vi "Complex Trigger Add Trigger.vi"(7 "Threshold S1/S2":u16(ring) items=["S1", "S2"], 8 "error in (no error)":errorcluster, 9 "Positive or negative (edge or level)":u16(ring) items=["Positive", "Negative"], 10 "Channel":u16(ring) items=["A1", "A2", "A3", "A4", "A5", "A6", "A7", "A8", "A9", "A10", "A11", "A12", "A13", "A14", "A15", "A16", "A17", "A18", "A19", "A20", "B1", "B2", "B3", "B4", "B5", "B6", "B7", "B8", "B9", "B10", "B11", "B12", "B13", "B14", "B15", "B16", "B17", "B18", "B19", "B20", "C1", "C2", "C3", "C4", "C5", "C6", "C7", "C8", "C9", "C10", "C11", "C12", "C13", "C14", "C15", "C16", "C17", "C18", "C19", "C20", "D1", "D2", "D3", "D4", "D5", "D6", "D7", "D8", "D9", "D10", "D11", "D12", "D13", "D14", "D15", "D16", "D17", "D18", "D19", "D20", "E1", "E2", "E3", "E4", "E5", "E6", "E7", "E8", "E9", "E10", "E11", "E12", "E13", "E14", "E15", "E16", "E17", "E18", "E19", "E20", "F1", "F2", "F3", "F4", "F5", "F6", "F7", "F8", "F9", "F10", "F11", "F12", "F13", "F14", "F15", "F16", "F17", "F18", "F19", "F20", "G1", "G2", "G3", "G4", "G5", "G6", "G7", "G8", "G9", "G10", "G11", "G12", "G13", "G14", "G15", "G16", "G17", "G18", "G19", "G20", "H1", "H2", "H3", "H4", "H5", "H6", "H7", "H8", "H9", "H10", "H11", "H12", "H13", "H14", "H15", "H16", "H17", "H18", "H19", "H20", "I1", "I2", "I3", "I4", "I5", "I6", "I7", "I8", "I9", "I10", "I11", "I12", "I13", "I14", "I15", "I16", "I17", "I18", "I19", "I20", "J1", "J2", "J3", "J4", "J5", "J6", "J7", "J8", "J9", "J10", "J11", "J12", "J13", "J14", "J15", "J16", "J17", "J18", "J19", "J20", "K1", "K2", "K3", "K4", "FA1", "FA2", "FA3", "FA4", "FB1", "FB2", "FB3", "FB4", "FC1", "FC2", "FC3", "FC4", "FD1", "FD2", "FD3", "FD4", "FE1", "FE2", "FE3", "FE4", "FF1", "FF2", "FF3", "FF4", "FG1", "FG2", "FG3", "FG4", "FH1", "FH2", "FH3", "FH4", "FI1", "FI2", "FI3", "FI4", "FJ1", "FJ2", "FJ3", "FJ4"], 11 "VISA resource name":refnum<visa-resource-name>) -> (0 "error out":errorcluster, 3 "VISA resource name out":refnum<visa-resource-name>)   [LabVIEW 2017, in "Sefram DAS220.lvlib"]
doc: "Add a trigger condition for complex (multiple) trigger."
uses:
  <instrlib>/Sefram DAS220/Sefram DAS220.lvlib
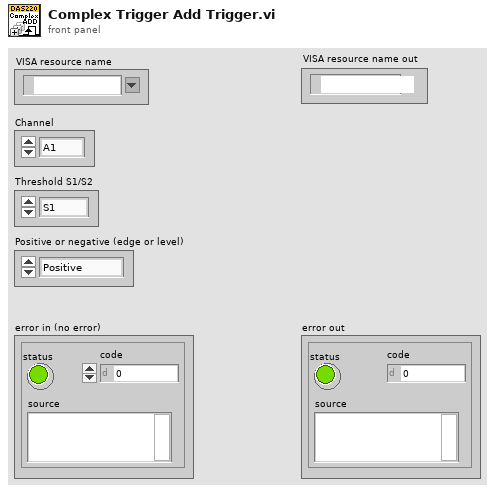
[diagram p1: front panel]
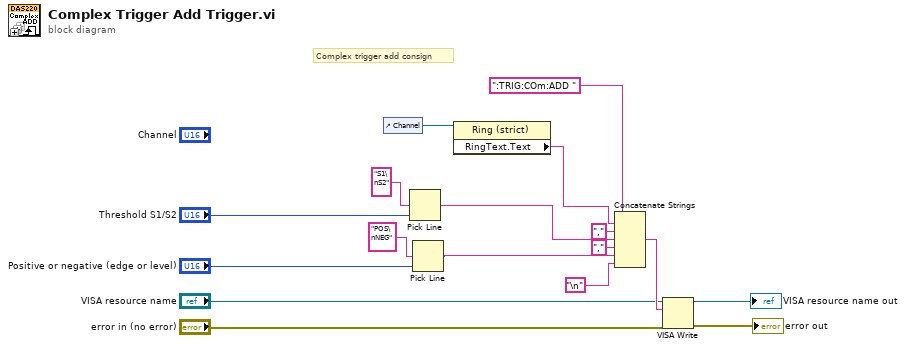
[diagram p0: block diagram]
diagram:
  # "Complex trigger add consign"
  n1 = control-ref of="Channel"() -> (w1:refnum<vi>)
  n2 = Pick Line(multi-line string="S1\nS2", line index="Threshold S1/S2") -> (output string=w7:string)  [unwired: 1 in]
  n3 = Pick Line(multi-line string="POS\nNEG", line index="Positive or negative (edge or level)") -> (output string=w4:string)  [unwired: 1 in]
  n4 = property class="Ring (strict)"(reference=w1) -> ("RingText.Text"=w9:string)  [unwired: 1 in, 2 out]
  n5 = Concatenate Strings(":TRIG:COm:ADD " ("string"), w9, "," ("string"), w7, "," ("string"), w4, "\n") -> (w17:string)
  n6 = VISA Write(VISA resource name="VISA resource name", write buffer=w17, error in (no error)="error in (no error)") -> (VISA resource name out=→"VISA resource name out":refnum<visa-resource-name>, error out=→"error out":errorcluster)  [unwired: 1 out]
